vi "CopyLibraryNoShift.vi"(7 "app":refnum<vi>, 8 "error in (no error)":errorcluster, 9 "new library name":string, 10 "new folder":path, 11 "source library path":path) -> (0 "error out":errorcluster, 2 "copied library":refnum<vi>, 3 "copied library path":path)   [LabVIEW 2022 SP3, in "FlexBlocks Support.lvlib"]
uses:
  FlexBlocks Support.lvlib
  <resource>/ChannelSupport/_ChannelScriptingSupport/_ChannelScriptingSupport.lvlib
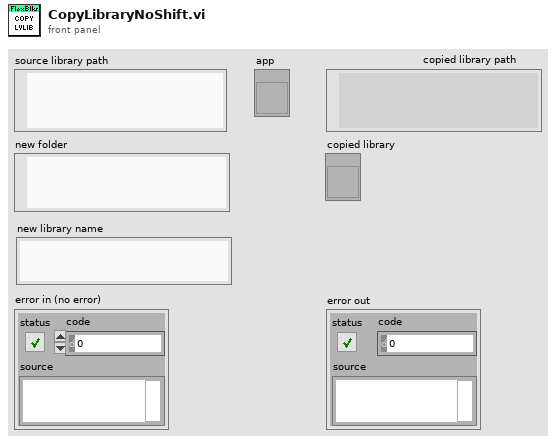
[diagram p1: front panel]
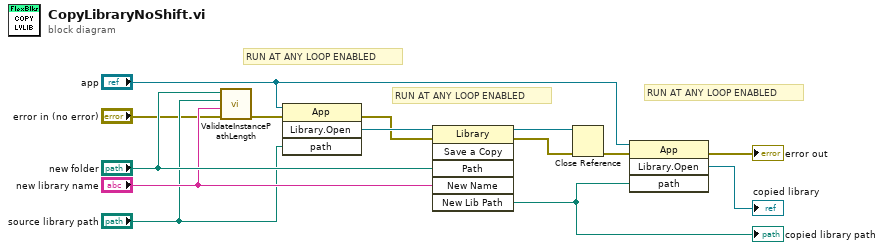
[diagram p0: block diagram]
diagram:
  # "RUN AT ANY LOOP ENABLED"
  # "RUN AT ANY LOOP ENABLED"
  # "RUN AT ANY LOOP ENABLED"
  n1 = call <resource>:"ValidateInstancePathLength.vi"("error in (no error)"="error in (no error)", "new library name"="new library name", "source library path"="source library path", "new folder"="new folder") -> ("error out"=w3:errorcluster)  [unwired: 7 in]
  n2 = invoke class="App" method="Library.Open"(reference="app", error in=w3, "path"="source library path") -> (error out=w11:errorcluster, "Open Library"=w12:refnum<vi>)  [unwired: 1 in, 2 out]
  n3 = invoke class="Library" method="Save a Copy"(reference=w12, error in=w11, "Path"="new folder", "New Name"="new library name") -> (reference out=w14:refnum<vi>, error out=w13:errorcluster, "New Lib Path"=w8:path)  [unwired: 2 in, 3 out]
  "copied library path" <- w8
  n4 = Close Reference(reference=w14, error in (no error)=w13) -> (error out=w10:errorcluster)
  n5 = invoke class="App" method="Library.Open"(reference="app", error in=w10, "path"=w8) -> (error out=→"error out":errorcluster, "Open Library"=→"copied library":refnum<vi>)  [unwired: 1 in, 2 out]
